vi "User LED Command.vi"(9 "LED Number":u8, 10 "LED Commands":T1=enum."Disable", 11 "Port":i32) -> (0 "Error":errorcluster, 3 "Port":i32)   [LabVIEW 2010]
uses:
  LED Commands.ctl
  Command Classes.ctl
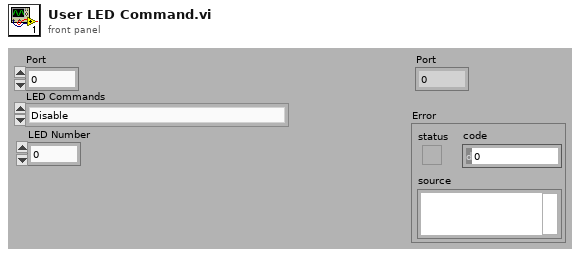
[diagram p1: front panel]
types:
  T1 = typedef "LED Commands.ctl" = enum16{"Enable", "Disable", "Toggle"}
  T2 = typedef "Command Classes.ctl" = enum8{"User Led", "Protocol"}
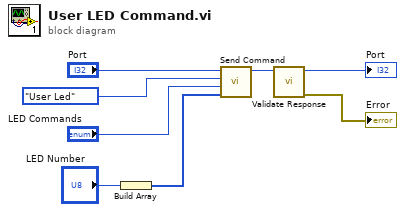
[diagram p0: block diagram]
diagram:
  n1 = Build Array("LED Number") -> (w4:u8[])
  n2 = call "Send Command.vi"("Parameters"=w4, "Command Type"="LED Commands", "Command Class"=Command_Classes."User Led", "Port"="Port") -> ("Port"=w3:i32)  [unwired: 7 in]
  n3 = call "Validate Response.vi"("Port"=w3) -> ("Error"=→"Error":errorcluster, "Port"=→"Port":i32)  [unwired: 9 in]
